vi "Initialize Data.vi"(8 "error in (no error)":errorcluster, 9 "data version":T1, 10 "data":string, 11 "Core Plugins Configuration in":refnum<class "Core Plugins Configuration.lvclass">) -> (0 "error out":errorcluster, 3 "Core Plugins Configuration out":refnum<class "Core Plugins Configuration.lvclass">)   [LabVIEW 2017, in "DSF Core.lvlib" / "Core Plugins Configuration.lvclass"]
uses:
  Core Plugins Configuration.lvclass
  Typedefs/DSF Version Info.ctl
  Core Plugins Configuration.lvclass/Core Plugins Configuration.ctl
  DSF Core.lvlib
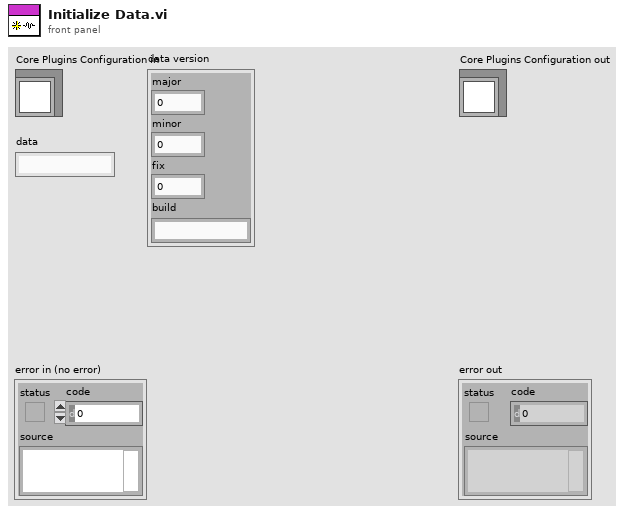
[diagram p1: front panel]
types:
  T1 = typedef "DSF Core.lvlib/DSF Version Info.ctl" = cluster{"major":i32, "minor":i32, "fix":i32, "build":string}
  T2 = cluster{"name":string, "components":string[], "cycle timing":cluster{"priority":u64, "decimation":u64, "offset":u64}}[]
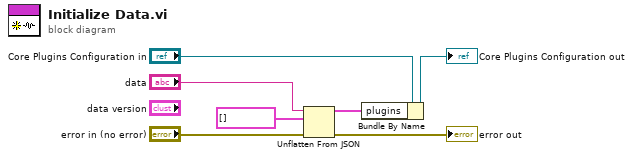
[diagram p0: block diagram]
diagram:
  n1 = Unflatten From JSON(JSON string="data", type and defaults=T2 [] ("plugins"), error in (no error)="error in (no error)") -> (value=w1:T2, error out=→"error out":errorcluster)  [unwired: 4 in]
  n2 = Bundle By Name(cluster="Core Plugins Configuration in", "plugins"=w1) -> (→"Core Plugins Configuration out":refnum<class "Core Plugins Configuration.lvclass">)
